vi "OpenCL Error.vi"(8 "error in (no error)":errorcluster) -> (0 "error out":errorcluster)   [LabVIEW 2014]
uses:
  OpenCL/OpenCL States.ctl
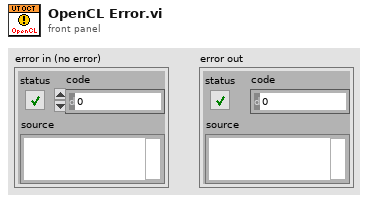
[diagram p1: front panel]
types:
  T1 = typedef "OpenCL States.ctl" = enum16{"Allocate Memory", "Get U16 Memory Dimension", "Compile Kernels", "Create Device", "Write", "Read", "Operate", "Delete Memory", "Delete"}
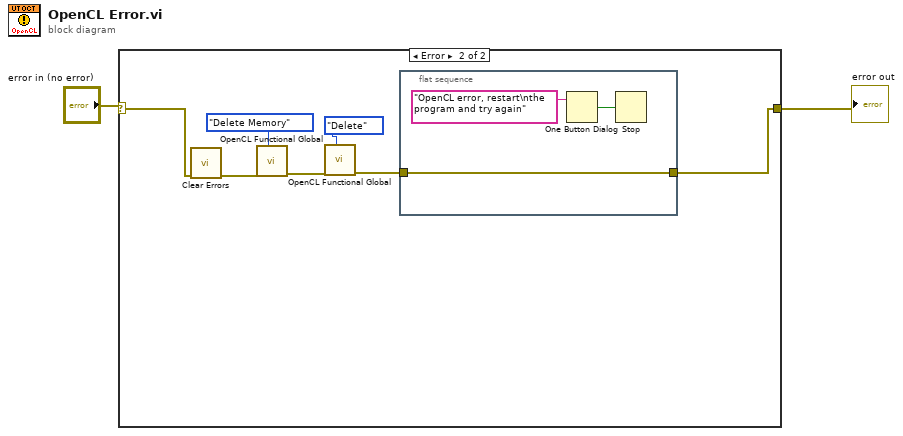
[diagram p0: block diagram]
diagram:
  n1 = case shown="Error" "error in (no error)" {
    selector: "error in (no error)" -> [w3 w6]
    tunnel: [w3 w4] -> w2
    frame No Error {
    }
    frame Error {
      n2 = call <vilib>:"Clear Errors.vi"("error in (no error)"=w6) -> ("error out"=w7:errorcluster)  [unwired: 5 in, 1 out]
      n3 = call "OpenCL Functional Global.vi"("States"=OpenCL_States."Delete Memory", "Error In"=w7) -> ("Error Out"=w9:errorcluster)  [unwired: 6 in, 3 out]
      n4 = call "OpenCL Functional Global.vi"("States"=OpenCL_States."Delete", "Error In"=w9) -> ("Error Out"=w5:errorcluster)  [unwired: 6 in, 3 out]
      n5 = flat-sequence {
        tunnel: [w12] -> w4
        tunnel: w5 -> [w12]
        frame #0 {
          n6 = One Button Dialog(message="OpenCL error, restart\nthe program and try again") -> (true=w11:bool)  [unwired: 1 in]
          n7 = Stop(stop? (T)=w11) -> ()
        }
      }
    }
  }
  "error out" <- w2
